vi "EX 2-1Blink.vi"   [LabVIEW 2011]
doc: "An example that reads a user selectable analog input pin on the Arduino."
uses:
  <vilib>/LabVIEW Interface for Arduino/Type Defs/Board Type.ctl
  <vilib>/LabVIEW Interface for Arduino/Type Defs/Connection Type.ctl
  <vilib>/LabVIEW Interface for Arduino/Type Defs/Pin Mode.ctl
  <vilib>/LabVIEW Interface for Arduino/LabVIEW Interface for Arduino.lvlib
types:
  T1 = typedef "LabVIEW Interface for Arduino.lvlib/Pin Mode.ctl" = enum8{"Input", "Output"}
  T2 = typedef "LabVIEW Interface for Arduino.lvlib/Connection Type.ctl" = enum8{"USB / Serial", "XBEE", "BlueSmirf (Bluetooth)"}
  T3 = typedef "LabVIEW Interface for Arduino.lvlib/Board Type.ctl" = enum16{"Uno", "Dimuelanove w/Atmega 328", "Mega 2560"}
  T4 = typedef "LabVIEW Interface for Arduino.lvlib/Arduino Resource.ctl" = cluster{"VISA resource":refnum<visa-resource-name>, "Board Type":T3, "Connection Type":enum8{"USB / Serial"}, "Bytes Per Packet (15)":u8}
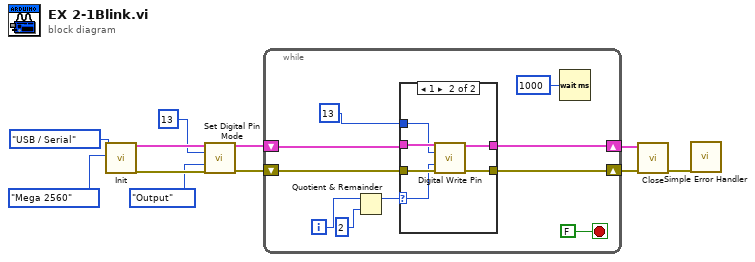
[diagram p0: block diagram]
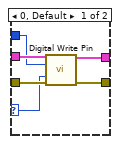
[diagram p2: hidden frame]
diagram:
  n1 = call <vilib>:"Init.vi"("Board Type (Uno)"=Board_Type."Mega 2560", "Connection Type (USB/Serial)"=Connection_Type."USB / Serial") -> ("Arduino Resource"=w6:T4, "error out"=w3:errorcluster)  [unwired: 16 in]
  n2 = call <vilib>:"Set Digital Pin Mode.vi"("Arduino Resource"=w6, "Digital I/O Pin"=u8 13, "Pin Mode (Input)"=Pin_Mode."Output", "error in"=w3) -> ("Arduino Resource"=w5:T4, "error out"=w4:errorcluster)  [unwired: 10 in]
  n3 = while {
    shift-right: [w20] -> w11
    shift-left: w5 -> [w13]
    shift-right: [w19] -> w10
    shift-left: w4 -> [w12]
    i -> [w16]
    stop <- FALSE stop-if-true
    n4 = Quotient & Remainder(x=w16, y=2) -> (x-y*floor(x/y)=w14:i32)  [unwired: 1 out]
    n5 = case shown="1" w14 {
      selector: w14 -> [w22 w28]
      tunnel: w13 -> [w25 w33]
      tunnel: [w24 w32] -> w20
      tunnel: [w26 w31] -> w19
      tunnel: w12 -> [w27 w30]
      tunnel: u8 13 ("Digital I/O Pin") -> [w23 w29]
      frame 0, Default {
        n6 = call <vilib>:"Digital Write Pin.vi"("Arduino Resource"=w25, "Digital I/O Pin (0)"=w23, "Value (0)"=w22, "error in"=w27) -> ("Arduino Resource"=w24:T4, "error out"=w26:errorcluster)  [unwired: 10 in]
      }
      frame 1 {
        n7 = call <vilib>:"Digital Write Pin.vi"("Arduino Resource"=w33, "Digital I/O Pin (0)"=w29, "Value (0)"=w28, "error in"=w30) -> ("Arduino Resource"=w32:T4, "error out"=w31:errorcluster)  [unwired: 10 in]
      }
    }
    n8 = Wait (ms)(milliseconds to wait=u32 1000) -> ()  [unwired: 1 out]
  }
  n9 = call <vilib>:"Close.vi"("Arduino Resource"=w11, "error in"=w10) -> ("error out"=w9:errorcluster)  [unwired: 13 in]
  n10 = call <vilib>:"Simple Error Handler.vi"("error in (no error)"=w9) -> ()  [unwired: 4 in, 5 out]
